vi "Read_Resource.vi"(8 "error in (no error)":errorcluster, 11 "VISA Refnum in":refnum<visa-resource-name>) -> (0 "error out":errorcluster, 2 "read buffer":string, 3 "VISA Refnum out":refnum<visa-resource-name>)   [LabVIEW 2014]
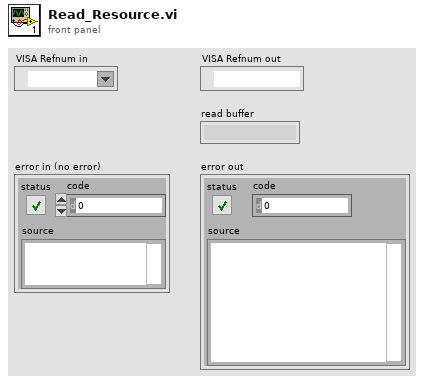
[diagram p1: front panel]
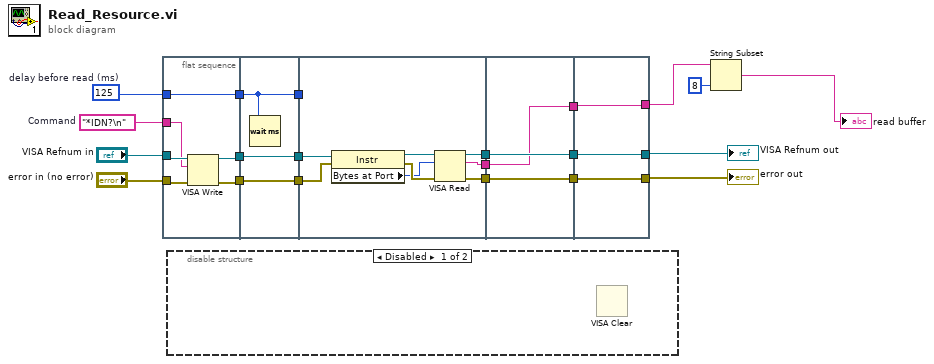
[diagram p0: block diagram]
diagram:
  w21 = u32 125  # delay before read (ms)
  w17 = "*IDN?\n"  # Command
  n1 = flat-sequence {
    tunnel: w21 -> [w27]
    tunnel: [w27] -> w20
    tunnel: "VISA Refnum in" -> [w26]
    tunnel: "error in (no error)" -> [w25]
    tunnel: w17 -> [w22]
    tunnel: [w23] -> w12
    tunnel: [w24] -> w10
    tunnel: w20 -> [w30]
    tunnel: [w30] -> w14
    tunnel: [w29] -> w13
    tunnel: w12 -> [w29]
    tunnel: [w28] -> w11
    tunnel: w10 -> [w28]
    tunnel: [w35] -> w9
    tunnel: [w34] -> w7
    tunnel: [w33] -> w5
    tunnel: w14 -> [_]
    tunnel: w13 -> [w32]
    tunnel: w11 -> [w31]
    tunnel: w9 -> [w41]
    tunnel: [w41] -> w8
    tunnel: w7 -> [w40]
    tunnel: [w40] -> w6
    tunnel: w5 -> [w39]
    tunnel: [w39] -> w4
    tunnel: w8 -> [w43]
    tunnel: w6 -> [w42]
    tunnel: w4 -> [w44]
    tunnel: [w43] -> w15
    tunnel: [w42] -> w16
    tunnel: [w44] -> w3
    frame #0 {
      n2 = VISA Write(VISA resource name=w26, write buffer=w22, error in (no error)=w25) -> (VISA resource name out=w23:refnum<visa-resource-name>, error out=w24:errorcluster)  [unwired: 1 out]
    }
    frame #1 {
      n3 = Wait (ms)(milliseconds to wait=w30) -> ()  [unwired: 1 out]
    }
    frame #2 {
      n4 = property class="Instr"(reference=w32, error in=w31) -> (reference out=w38:refnum<visa-resource-name>, error out=w37:errorcluster, "Bytes at Port"=w36:u32)
      n5 = VISA Read(VISA resource name=w38, byte count=w36, error in (no error)=w37) -> (VISA resource name out=w34:refnum<visa-resource-name>, read buffer=w33:string, error out=w35:errorcluster)  [unwired: 1 out]
    }
    frame #3 {
    }
    frame #4 {
    }
  }
  n6 = disable-structure shown="Disabled" {
    frame Disabled {
      n7 = VISA Clear() -> ()  [unwired: 2 in, 2 out]
    }
    frame Enabled {
    }
  }
  n8 = String Subset(string=w3, length (rest)=8 ("length (rest)")) -> (substring=→"read buffer":string)  [unwired: 1 in]
  "error out" <- w15
  "VISA Refnum out" <- w16
